vi "DefendAreaTactic.vi"(6 "Number of Defenders\nWithout Duelist":i32, 8 "error in (no error)":errorcluster, 9 "Robot":refnum<class "Robot.lvclass">, 10 "Game in":refnum<class "Game.lvclass">, 11 "DefendAreaTactic in":refnum<class "DefendAreaTactic.lvclass">) -> (0 "error out":errorcluster, 2 "Robot out":refnum<class "Robot.lvclass">, 3 "DefendAreaTactic out":refnum<class "DefendAreaTactic.lvclass">)   [LabVIEW 2023, in "DefendAreaTactic.lvclass"]
uses:
  DefendAreaTactic.lvclass
  Robot_class/Robot.lvclass
  Game_class/Game.lvclass
  TestTactic_class/States.ctl
  Robot_class/tactics.ctl
  Tactic_class/Tactic.lvclass/Tactic.ctl
  Robot_class/Robot.lvclass/Robot.ctl
  Tactic_class/Read Skillbook.vi
  Robot_class/Write tactic.vi
  Skillbook_class/Skillbook.lvclass
  DefendAreaSkill_class/DefendAreaSkill.lvclass
panel:
  out "x .or. y?":bool
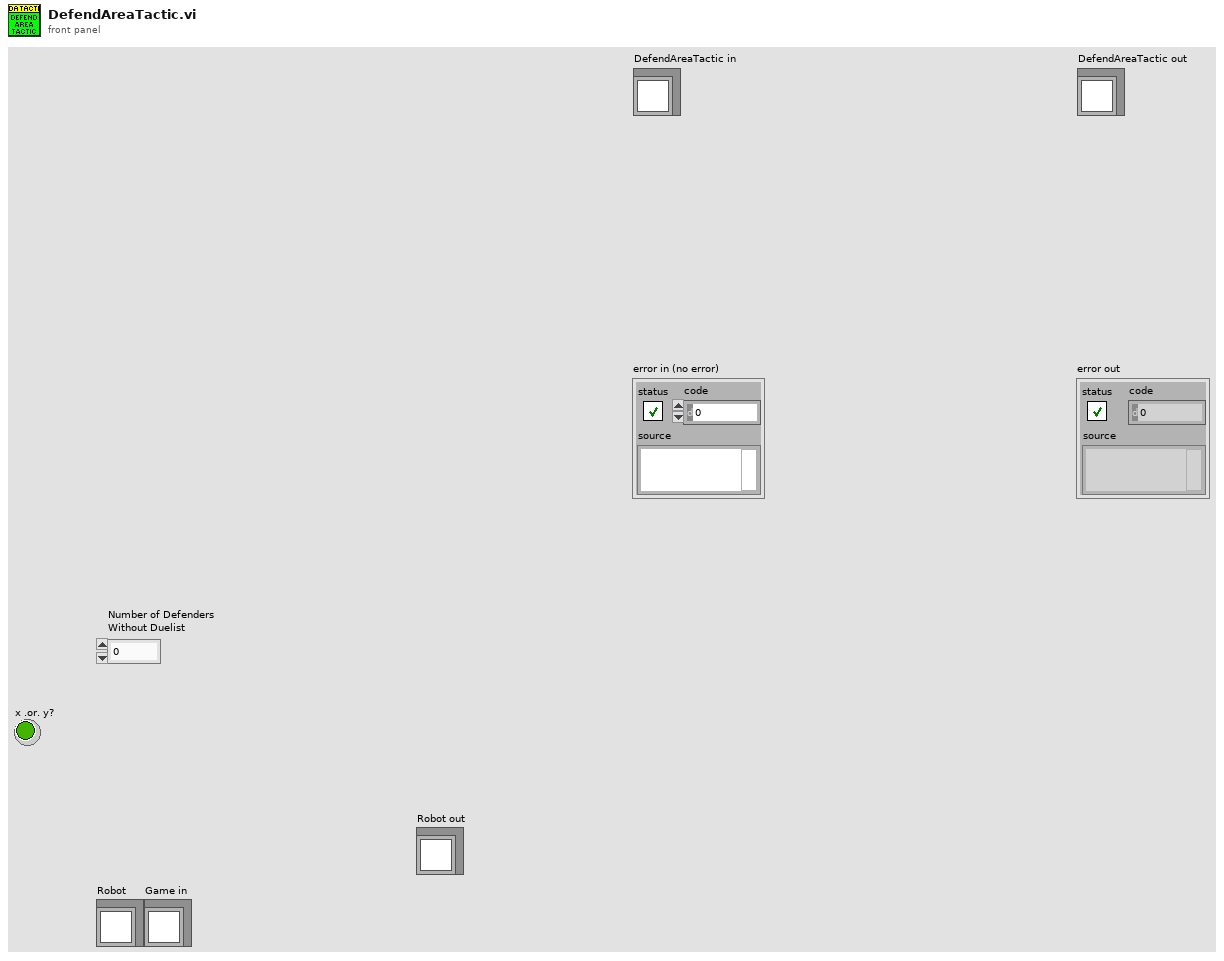
[diagram p1: front panel]
types:
  T1 = typedef "tactics.ctl" = enum16{"ReceivePassInFuturePoint", "Roller", "PrepareRollToPassRollerGoTo", "PrepareRollToPassReceiverGoTo", "WaitRoll", "PositionToRoll", "PenaltyAttacker", "PassObserver", "PenaltyDefense", "TableReceiverTactic", "Test", "DefendGoal", "Marker", "FollowAttacker", "DefendArea", "Shoot", "AttackerAimGoal", "AttackerBallOutOfField", "AttackerBlock", "AttackerStop", "Duelist", "Halt", "ZigZag", "GoTo", "Timeout", "KickToPassReceiver", "PositionToReceivePass", "DefendAreaVSS", "DefendGoalVSS", "KickVSS", "AttackVSS", "DispBallVSS", "PenaltyAttackVSS", "WaitPass"}
  T2 = typedef "States.ctl" = enum16{"State 1", "Exit"}
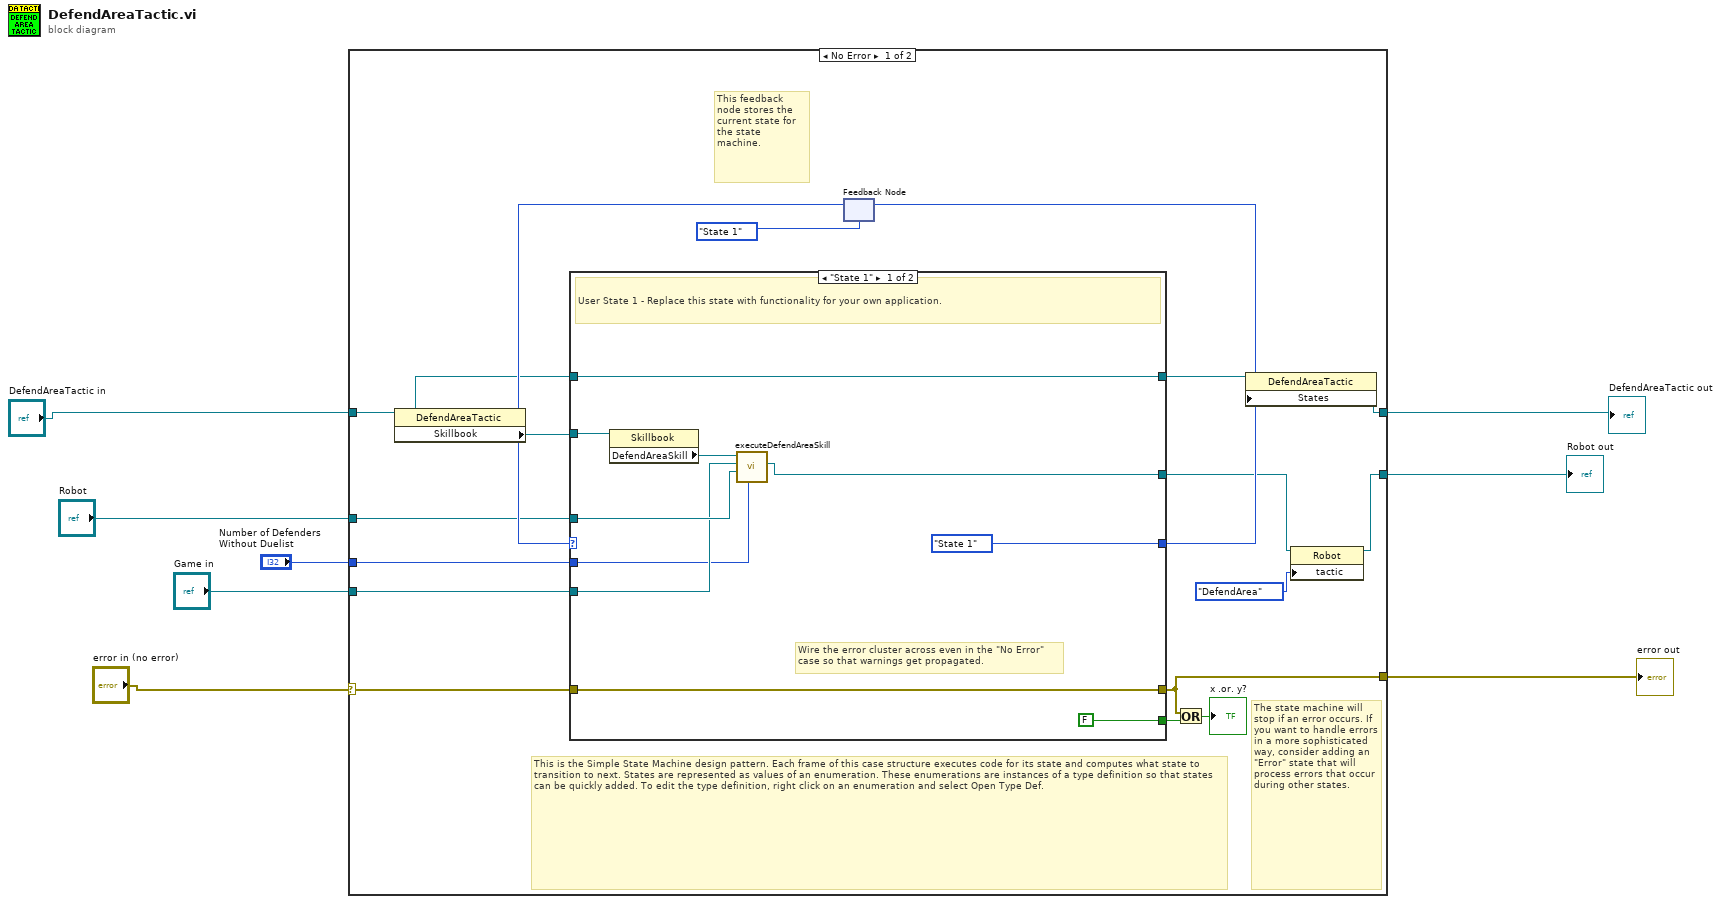
[diagram p0: block diagram]
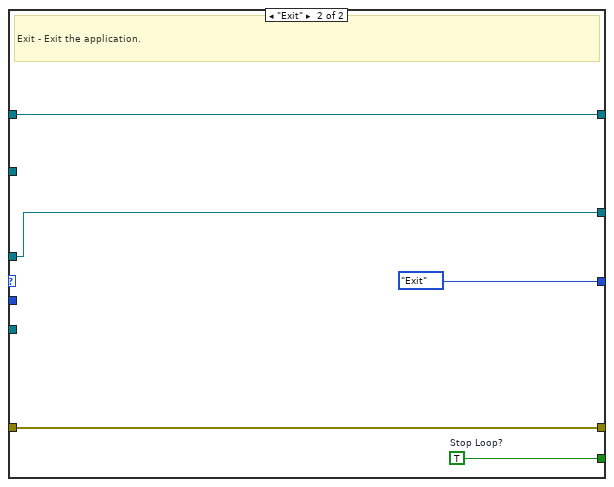
[diagram p2: hidden frame]
diagram:
  n1 = case shown="No Error" "error in (no error)" {
    selector: "error in (no error)" -> [w22 w43]
    tunnel: [w21 w43] -> w3
    tunnel: [w15 w42] -> w2
    tunnel: "DefendAreaTactic in" -> [w18 w42]
    tunnel: "Robot" -> [w19 w41]
    tunnel: [w9 w41] -> w7
    tunnel: "Game in" -> [w13 _]
    tunnel: "Number of Defenders\nWithout Duelist" -> [w12 _]
    frame No Error {
      # "The state machine will stop if an error occurs. If you want to handle errors in a more sophisticated way, consider adding an \"Error\" state that will process errors that occur during other states."
      # "This feedback node stores the current state for the state machine."
      # "This is the Simple State Machine design pattern. Each frame of this case structure executes code for its state and computes what state to transition to next. States are represented as values of an enumeration. These enumerations are instances of a type definition so that states can be quickly added. To edit the type definition, right click on an enumeration and select Open Type Def."
      # "Wire the error cluster across even in the \"No Error\"\ncase so that warnings get propagated."
      n2 = property class="DefendAreaTactic"(reference=w18) -> ("Skillbook"=w17:refnum<class "Skillbook.lvclass">)  [unwired: 1 in, 2 out]
      n3 = feedback #1(States."State 1" ("States")) -> (w23:T2)
      n4 = case shown="\"State 1\"" w23 {
        tunnel: [States."State 1" ("States") States."Exit" ("States")] -> w14
        tunnel: [FALSE ("Stop Loop?") w40] -> w25
        tunnel: w22 -> [w34 w39]
        tunnel: [w34 w39] -> w21
        tunnel: w17 -> [w32 _]
        tunnel: w19 -> [w29 w37]
        tunnel: [w28 w37] -> w10
        tunnel: [w31 w36] -> w16
        tunnel: w18 -> [w31 w36]
        tunnel: w13 -> [w27 _]
        tunnel: w12 -> [w26 _]
        frame "State 1" {
          # "User State 1 - Replace this state with functionality for your own application."
          n5 = property class="Skillbook"(reference=w32) -> ("DefendAreaSkill"=w30:refnum<class "DefendAreaSkill.lvclass">)  [unwired: 1 in, 2 out]
          n6 = call "executeDefendAreaSkill.vi"("Number of Defenders\nWithout Duelist"=w26, "Robot in"=w29, "Game"=w27, "DefendAreaSkill in"=w30) -> ("Robot out"=w28:refnum<class "Robot.lvclass">)  [unwired: 5 in, 2 out]
        }
        frame "Exit" {
          w40 = TRUE  # Stop Loop?
          # "Exit - Exit the application."
        }
      }
      n7 = feedback-in #1(w14) -> ()
      n8 = Or(x=w21, y=w25) -> (x .or. y?=→"x .or. y?":bool)
      n9 = property class="DefendAreaTactic"(reference=w16, "States"=w14) -> (reference out=w15:refnum<class "DefendAreaTactic.lvclass">)  [unwired: 1 in, 1 out]
      n10 = property class="Robot"(reference=w10, "tactic"=tactics."DefendArea") -> (reference out=w9:refnum<class "Robot.lvclass">)  [unwired: 1 in, 1 out]
    }
    frame Error {
    }
  }
  "error out" <- w3
  "DefendAreaTactic out" <- w2
  "Robot out" <- w7
